vi "Sub Initialize.vi"(8 "error in (no error)":errorcluster, 11 "Measure Object in":refnum<class "VI Server Recorder.lvclass">) -> (0 "error out":errorcluster, 2 "Initialize Result":refnum<class "Acquired Result.lvclass">, 3 "Measure Object out":refnum<class "VI Server Recorder.lvclass">)   [LabVIEW 2019, in "VI Server Recorder.lvclass"]
uses:
  VI Server Recorder.lvclass
  C:/GitHub/LabActor/Worker/Worker.lvclass
  NHMFL_Core/Libraries/Instruments/Results/Acquired Result/Acquired Result.lvclass
  NHMFL_Core/Libraries/Instruments/Results/Start Stream Result/Start Stream Result.lvclass
  C:/GitHub/NHMFL_Core/Libraries/Instruments/Results/Acquired Result/Acquired Result.lvclass
  Worker/Worker.lvclass/Worker.ctl
  NHMFL_Core/Libraries/Instruments/Results/Start Stream Result/Start Stream Result.lvclass/Start Stream Result.ctl
  NHMFL_Core/Libraries/Instruments/Results/Acquired Result/Acquired Result.lvclass/Acquired Result.ctl
  Worker/Read Cycle period.vi
  NHMFL_Core/Libraries/Instruments/Results/Start Stream Result/Write dt.vi
  NHMFL_Core/Libraries/Instruments/Results/Acquired Result/Write Channels.vi
  NHMFL_Core/Libraries/Instruments/Results/Acquired Result/Write Group.vi
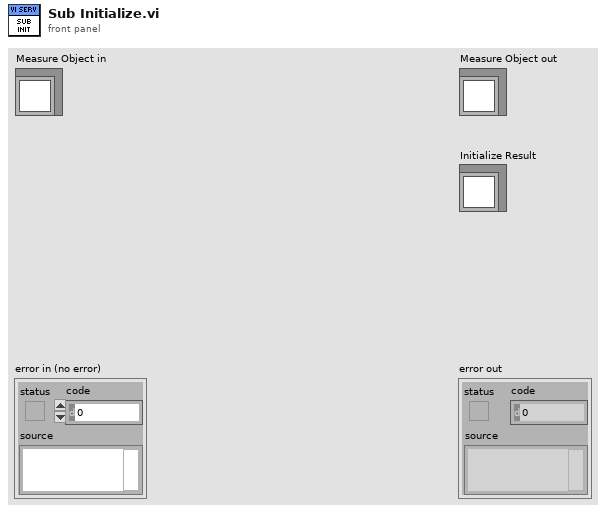
[diagram p1: front panel]
types:
  T1 = typedef "VI Server Configuration.ctl" = cluster{"Machine name (\"\":  open local reference)":string, "Port number (3363)":u16, "Control names":string[], "VI  name":string}
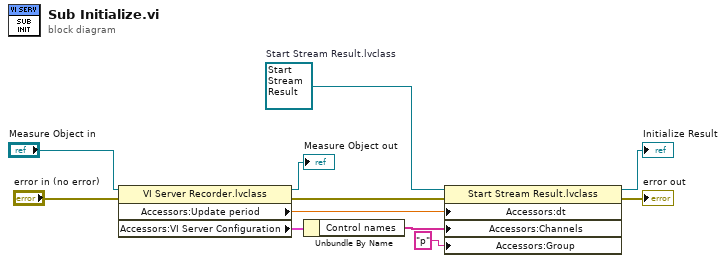
[diagram p0: block diagram]
diagram:
  w6 = refnum<class "Start Stream Result.lvclass"> refnum  # Start Stream Result.lvclass
  n1 = property class="VI Server Recorder.lvclass"(reference="Measure Object in", error in="error in (no error)") -> (reference out=→"Measure Object out":refnum<class "VI Server Recorder.lvclass">, error out=w3:errorcluster, "Accessors:Update period"=w10:dbl, "Accessors:VI Server Configuration"=w8:T1)
  n2 = Unbundle By Name(w8) -> ("Control names"=w7:string[])
  n3 = property class="Start Stream Result.lvclass"(reference=w6, error in=w3, "Accessors:dt"=w10, "Accessors:Channels"=w7, "Accessors:Group"="p" ("Group")) -> (reference out=→"Initialize Result":refnum<class "Start Stream Result.lvclass">, error out=→"error out":errorcluster)
